vi "FeedbackDecode_DEKACalibrate.vi"(3 "LoopCnt":i32, 4 "SensorsIn":T1={"Position"={"WriRot"=nan, "WriPitch"=nan, "IndFlex"=nan, "MRPFlex"=nan, "ThuRawPitch"=nan, "ThuRawYaw"=nan, "ThuYaw"=nan, "ThuPitch"=nan}, "Force"={"IndLat"=nan, "IndTip"=nan, "MidTip"=nan, "RinTip"=nan, "PinkyTip"=nan, "PalmDist"=nan, "PalmProx"=nan, "HandEdge"=nan, "HandDorsal"=nan, "ThuUlnar"=nan, "ThuRadial"=nan, "ThuTip"=nan, "ThuDorsal"=nan}}, 5 "Mode":enum16{"reset", "run"}(ring)) -> (0 "MSMSMvnt":dbl[](array[numeric]) min=-1.0 max=1.0, 1 "Status":bool, 2 "MinMax":dbl[][](array[numeric])=[[nan, nan, nan, nan, nan, nan, nan, nan, nan, nan, nan, nan, nan], [nan, nan, nan, nan, nan, nan, nan, nan, nan, nan, nan, nan, nan]])   [LabVIEW 2020]
panel:
  out "iMinMax":dbl[][](array[numeric])=[[nan, nan, nan, nan, nan, nan, nan, nan, nan, nan, nan, nan, nan], [nan, nan, nan, nan, nan, nan, nan, nan, nan, nan, nan, nan, nan]]
  out "BaseCnt":i32
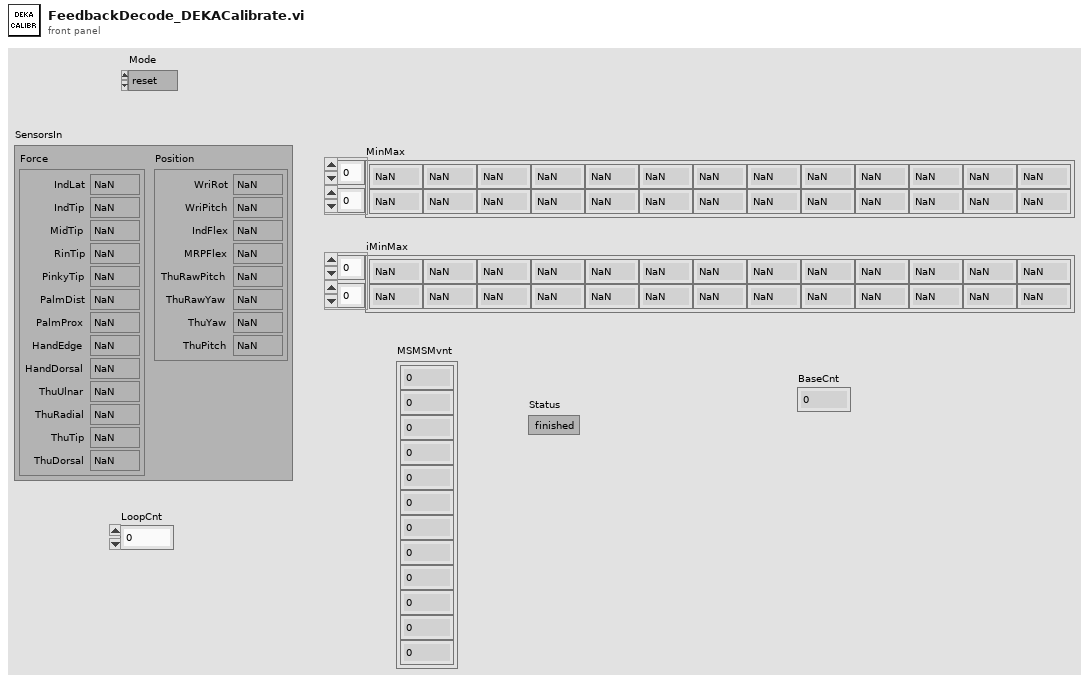
[diagram p1: front panel]
types:
  T1 = cluster{"Position":cluster{"WriRot":dbl, "WriPitch":dbl, "IndFlex":dbl, "MRPFlex":dbl, "ThuRawPitch":dbl, "ThuRawYaw":dbl, "ThuYaw":dbl, "ThuPitch":dbl}, "Force":cluster{"IndLat":dbl, "IndTip":dbl, "MidTip":dbl, "RinTip":dbl, "PinkyTip":dbl, "PalmDist":dbl, "PalmProx":dbl, "HandEdge":dbl, "HandDorsal":dbl, "ThuUlnar":dbl, "ThuRadial":dbl, "ThuTip":dbl, "ThuDorsal":dbl}}
  T2 = cluster{"IndLat":dbl, "IndTip":dbl, "MidTip":dbl, "RinTip":dbl, "PinkyTip":dbl, "PalmDist":dbl, "PalmProx":dbl, "HandEdge":dbl, "HandDorsal":dbl, "ThuUlnar":dbl, "ThuRadial":dbl, "ThuTip":dbl, "ThuDorsal":dbl}
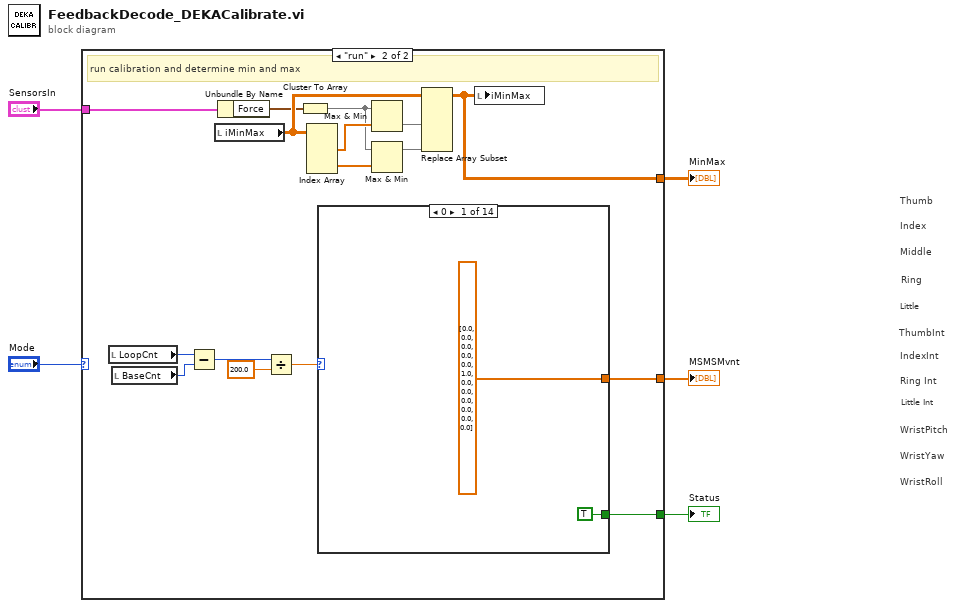
[diagram p0: block diagram]
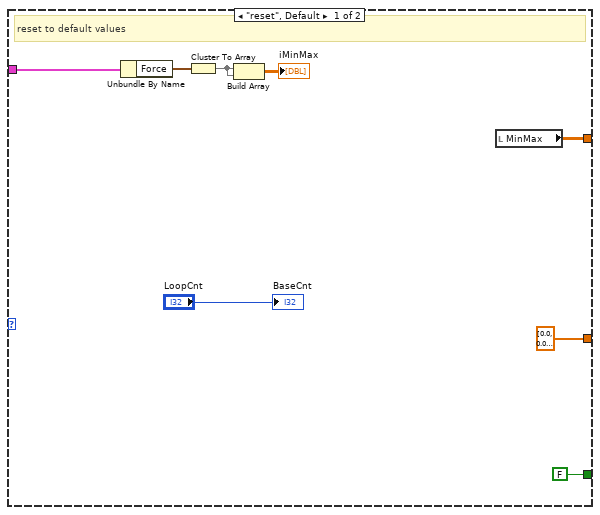
[diagram p2: hidden frame]
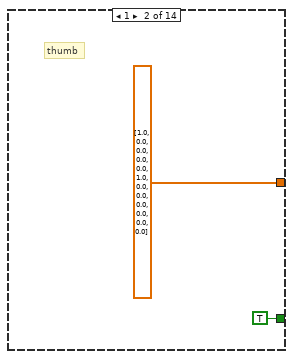
[diagram p3: hidden frame]
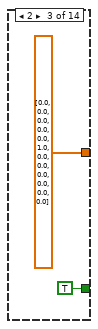
[diagram p4: hidden frame]
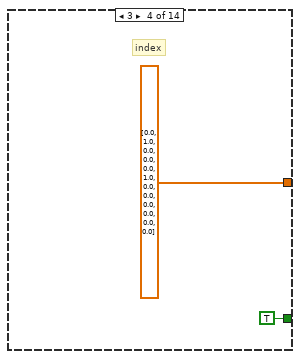
[diagram p5: hidden frame]
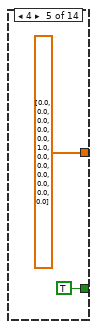
[diagram p6: hidden frame]
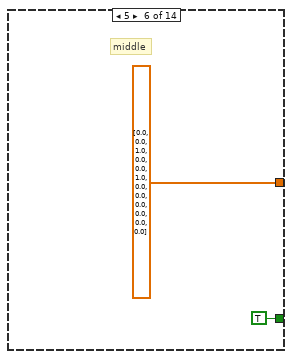
[diagram p7: hidden frame]
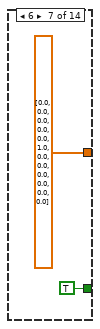
[diagram p8: hidden frame]
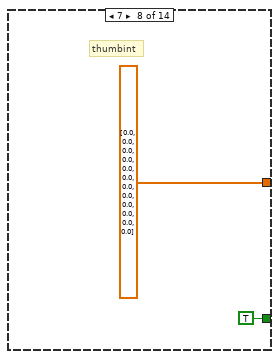
[diagram p9: hidden frame]
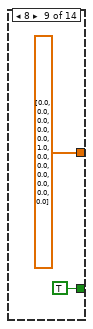
[diagram p10: hidden frame]
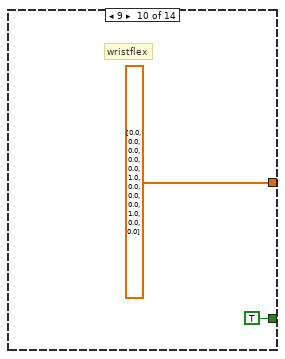
[diagram p11: hidden frame]
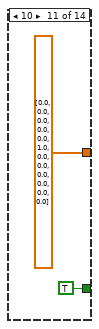
[diagram p12: hidden frame]
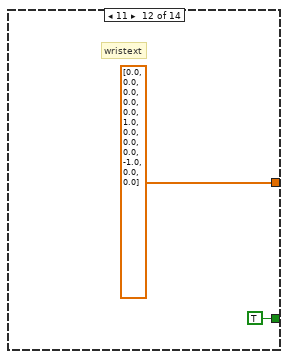
[diagram p13: hidden frame]
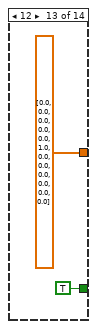
[diagram p14: hidden frame]
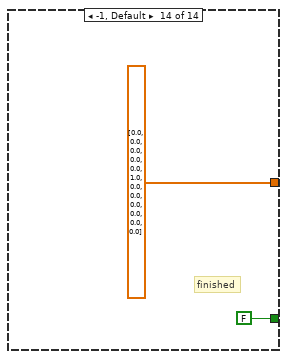
[diagram p15: hidden frame]
diagram:
  # "Little Int"
  # "WristRoll"
  # "WristYaw"
  # "WristPitch"
  # "Ring Int"
  # "IndexInt"
  # "ThumbInt"
  # "Little"
  # "Ring"
  # "Middle"
  # "Index"
  # "Thumb"
  n1 = case shown="\"run\"" "Mode" {
    tunnel: [dbl[] [0.0, 0.0, 0.0, 0.0, 0.0, 0.0, 0.0, 0.0, 0.0, 0.0, 0.0, 0.0] ("MSMSMvnt") w26] -> w5
    tunnel: "SensorsIn" -> [w7 w14]
    tunnel: [w10 w15] -> w2
    tunnel: [FALSE w23] -> w1
    frame "reset", Default {
      # "reset to default values"
      n2 = Unbundle By Name(w7) -> ("Force"=w9:T2)
      n3 = Cluster To Array(cluster=w9) -> (array=w8:dbl[])
      n4 = Build Array(w8, w8) -> (→"iMinMax":dbl[][])
      n5 = local read "MinMax"() -> (w10:dbl[][])
      "BaseCnt" <- "LoopCnt"
    }
    frame "run" {
      # "run calibration and determine min and max"
      n6 = local read "LoopCnt"() -> (w25:i32)
      n7 = local read "BaseCnt"() -> (w24:i32)
      n8 = Subtract(x=w25, y=w24) -> (x-y=w29:i32)
      n9 = local read "iMinMax"() -> (w20:dbl[][])
      n10 = Unbundle By Name(w14) -> ("Force"=w16:T2)
      n11 = Divide(x=w29, y=200.0) -> (x/y=w27:dbl)
      n12 = Cluster To Array(cluster=w16) -> (array=w17:dbl[])
      n13 = Index Array(array=w20) -> (element #1=w18:dbl[], element #2=w19:dbl[])  [unwired: 4 in]
      n14 = case shown="0" w27 {
        tunnel: [dbl[] [0.0, 0.0, 0.0, 0.0, 0.0, 1.0, 0.0, 0.0, 0.0, 0.0, 0.0, 0.0] ("MSMSMvnt") dbl[] [1.0, 0.0, 0.0, 0.0, 0.0, 1.0, 0.0, 0.0, 0.0, 0.0, 0.0, 0.0] ("MSMSMvnt") dbl[] [0.0, 0.0, 0.0, 0.0, 0.0, 1.0, 0.0, 0.0, 0.0, 0.0, 0.0, 0.0] ("MSMSMvnt") dbl[] [0.0, 1.0, 0.0, 0.0, 0.0, 1.0, 0.0, 0.0, 0.0, 0.0, 0.0, 0.0] ("MSMSMvnt") dbl[] [0.0, 0.0, 0.0, 0.0, 0.0, 1.0, 0.0, 0.0, 0.0, 0.0, 0.0, 0.0] ("MSMSMvnt") dbl[] [0.0, 0.0, 1.0, 0.0, 0.0, 1.0, 0.0, 0.0, 0.0, 0.0, 0.0, 0.0] ("MSMSMvnt") dbl[] [0.0, 0.0, 0.0, 0.0, 0.0, 1.0, 0.0, 0.0, 0.0, 0.0, 0.0, 0.0] ("MSMSMvnt") dbl[] [0.0, 0.0, 0.0, 0.0, 0.0, 0.0, 0.0, 0.0, 0.0, 0.0, 0.0, 0.0] ("MSMSMvnt") dbl[] [0.0, 0.0, 0.0, 0.0, 0.0, 1.0, 0.0, 0.0, 0.0, 0.0, 0.0, 0.0] ("MSMSMvnt") dbl[] [0.0, 0.0, 0.0, 0.0, 0.0, 1.0, 0.0, 0.0, 0.0, 1.0, 0.0, 0.0] ("MSMSMvnt") dbl[] [0.0, 0.0, 0.0, 0.0, 0.0, 1.0, 0.0, 0.0, 0.0, 0.0, 0.0, 0.0] ("MSMSMvnt") dbl[] [0.0, 0.0, 0.0, 0.0, 0.0, 1.0, 0.0, 0.0, 0.0, -1.0, 0.0, 0.0] ("MSMSMvnt") dbl[] [0.0, 0.0, 0.0, 0.0, 0.0, 1.0, 0.0, 0.0, 0.0, 0.0, 0.0, 0.0] ("MSMSMvnt") dbl[] [0.0, 0.0, 0.0, 0.0, 0.0, 1.0, 0.0, 0.0, 0.0, 0.0, 0.0, 0.0] ("MSMSMvnt")] -> w26
        tunnel: [TRUE TRUE TRUE TRUE TRUE TRUE TRUE TRUE TRUE TRUE TRUE TRUE TRUE FALSE] -> w23
        frame 0 {
        }
        frame 1 {
          # "thumb"
        }
        frame 2 {
        }
        frame 3 {
          # "index"
        }
        frame 4 {
        }
        frame 5 {
          # "middle"
        }
        frame 6 {
        }
        frame 7 {
          # "thumbint"
        }
        frame 8 {
        }
        frame 9 {
          # "wristflex"
        }
        frame 10 {
        }
        frame 11 {
          # "wristext"
        }
        frame 12 {
        }
        frame -1, Default {
          # "finished"
        }
      }
      n15 = Max & Min(x=w17, y=w18) -> (min(x,y)=w21:dbl[])  [unwired: 1 out]
      n16 = Max & Min(x=w17, y=w19) -> (max(x,y)=w22:dbl[])  [unwired: 1 out]
      n17 = Replace Array Subset(array=w20, new element #1=w21, new element #2=w22) -> (w15:dbl[][])  [unwired: 4 in]
      n18 = local write "iMinMax"(w15) -> ()
    }
  }
  "MSMSMvnt" <- w5
  "MinMax" <- w2
  "Status" <- w1
